vi "collector power.vi"(8 "error in":errorcluster) -> (0 "error out":errorcluster, 3 "Collector/Ejector power":dbl)   [LabVIEW 2015]
uses:
  Support/Global Objects.vi
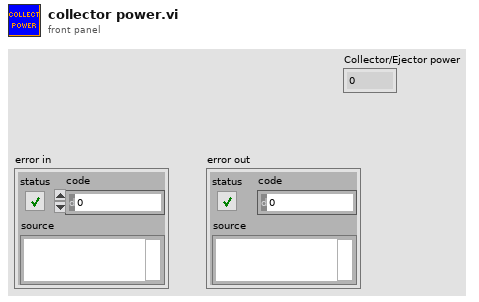
[diagram p1: front panel]
types:
  T1 = typedef "Teleop Commands.ctl" = cluster{"Throttle":dbl, "Turn":dbl, "Up Shift Commanded":bool, "Down Shift Commanded":bool, "Collect":bool, "Eject":bool}
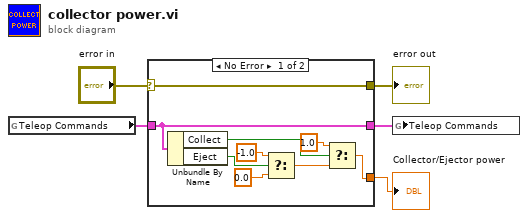
[diagram p0: block diagram]
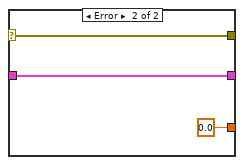
[diagram p2: hidden frame]
diagram:
  n1 = global read "Global Objects.vi" "Teleop Commands"() -> (w3:T1)
  n2 = case shown="No Error" "error in" {
    selector: "error in" -> [w13 w17]
    tunnel: [w13 w17] -> w4
    tunnel: [w14 w16] -> w2
    tunnel: w3 -> [w14 w16]
    tunnel: [w6 0.0 ("joyout")] -> w1
    frame No Error {
      n3 = Unbundle By Name(w14) -> ("Collect"=w11:bool, "Eject"=w10:bool)
      n4 = Select(t=-1.0, s=w10, f=0.0) -> (s? t:f=w7:dbl)
      n5 = Select(t=1.0, s=w11, f=w7) -> (s? t:f=w6:dbl)
    }
    frame Error {
    }
  }
  "error out" <- w4
  "Collector/Ejector power" <- w1
  n6 = global write "Global Objects.vi" "Teleop Commands"(w2) -> ()
